vi "FreqPeakFit.vi"(6 "error in (no error)":errorcluster, 8 "Peak fit width":i32=3 min=3, 9 "Waveform":waveform(dbl)={"t0"=timestamp(0.1098 s since 1904-01-01), "dt"=1e-07, "Y"=array[1000 elements], "attributes"=variant("Channel_name"=variant(string "CH1"), "NI_ChannelName"=variant(string "CH1"), "Total_points"=variant(i64 1200000))}) -> (0 "error out":errorcluster, 2 "Amplitude":dbl, 3 "PeakFreqOut":dbl)   [LabVIEW 2019]
uses:
  <vilib>/measure/mamon.llb/Waveform Peak Detection for 1 Chan.vi
  <vilib>/measure/NI_MAPro.lvlib
panel:
  out "Freq3":dbl
  out "Freq2":dbl
  out "Freq":dbl
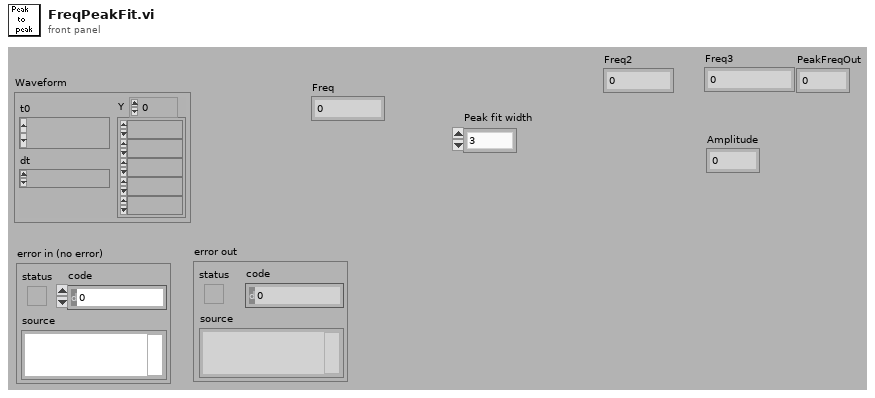
[diagram p1: front panel]
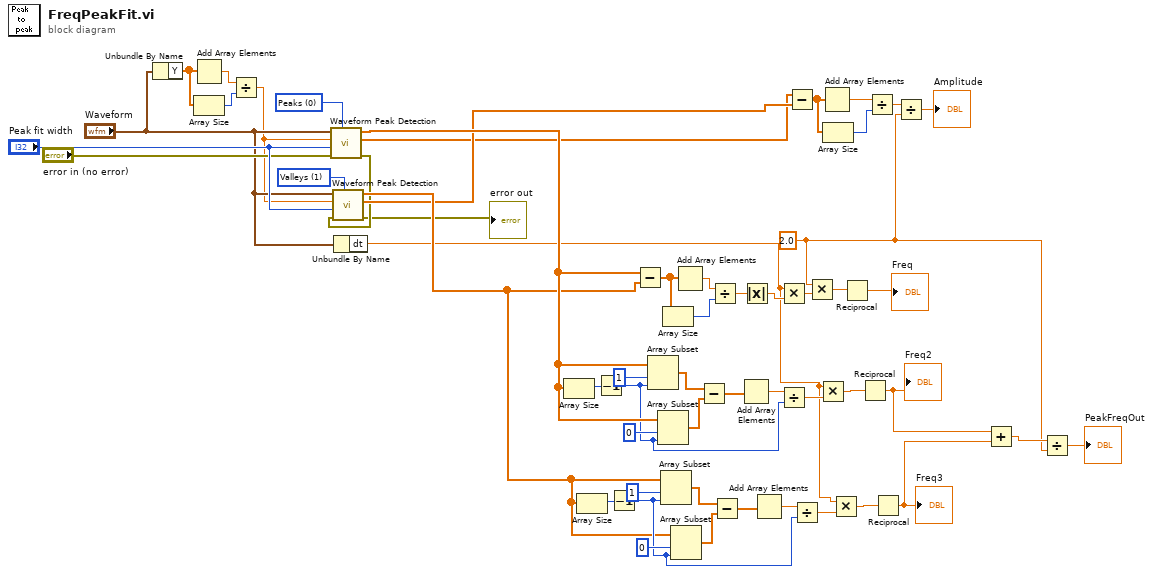
[diagram p0: block diagram]
diagram:
  w10 = u16 0 items=["Peaks", "Valleys"] ("peaks/valleys")
  w11 = 2.0
  w54 = u16 1 items=["Peaks", "Valleys"] ("peaks/valleys")
  n1 = Unbundle By Name("Waveform") -> ("Y"=w4:dbl[])
  n2 = Add Array Elements(numeric array=w4) -> (sum=w2:dbl)
  n3 = Array Size(array=w4) -> (size(s)=w3:i32)
  n4 = Divide(x=w2, y=w3) -> (x/y=w1:dbl)
  n5 = call-poly <vilib>:"Waveform Peak Detection.vi"("peaks/valleys"=w10, "error in"="error in (no error)", "width"="Peak fit width", "threshold"=w1, "Signal In"="Waveform") -> ("error out"=w7:errorcluster, "Amplitudes"=w14:dbl[], "Locations"=w39:dbl[])  [unwired: 2 in, 2 out]
  n6 = call-poly <vilib>:"Waveform Peak Detection.vi"("peaks/valleys"=w54, "error in"=w7, "width"="Peak fit width", "threshold"=w1, "Signal In"="Waveform") -> ("error out"=→"error out":errorcluster, "Amplitudes"=w18:dbl[], "Locations"=w19:dbl[])  [unwired: 2 in, 2 out]
  n7 = Unbundle By Name("Waveform") -> ("dt"=w9:dbl)
  n8 = Array Size(array=w39) -> (size(s)=w44:i32)
  n9 = Array Size(array=w19) -> (size(s)=w33:i32)
  n10 = Decrement(x=w44) -> (x-1=w36:i32)
  n11 = Decrement(x=w33) -> (x-1=w26:i32)
  n12 = Subtract(x=w39, y=w19) -> (x-y=w51:dbl[])
  n13 = Array Subset(array=w39, index=1, length=w36) -> (w41:dbl[])
  n14 = Array Subset(array=w39, index=0, length=w36) -> (w40:dbl[])
  n15 = Array Subset(array=w19, index=1, length=w26) -> (w30:dbl[])
  n16 = Array Size(array=w51) -> (size(s)=w49:i32)
  n17 = Array Subset(array=w19, index=0, length=w26) -> (w29:dbl[])
  n18 = Add Array Elements(numeric array=w51) -> (sum=w52:dbl)
  n19 = Subtract(x=w41, y=w40) -> (x-y=w38:dbl[])
  n20 = Divide(x=w52, y=w49) -> (x/y=w50:dbl)
  n21 = Subtract(x=w30, y=w29) -> (x-y=w28:dbl[])
  n22 = Add Array Elements(numeric array=w38) -> (sum=w37:dbl)
  n23 = Absolute Value(x=w50) -> (abs(x)=w48:dbl)
  n24 = Add Array Elements(numeric array=w28) -> (sum=w27:dbl)
  n25 = Multiply(x=w9, y=w48) -> (x*y=w47:dbl)
  n26 = Divide(x=w37, y=w36) -> (x/y=w35:dbl)
  n27 = Subtract(x=w14, y=w18) -> (x-y=w15:dbl[])
  n28 = Divide(x=w27, y=w26) -> (x/y=w25:dbl)
  n29 = Multiply(x=w11, y=w47) -> (x*y=w46:dbl)
  n30 = Multiply(x=w9, y=w35) -> (x*y=w34:dbl)
  n31 = Add Array Elements(numeric array=w15) -> (sum=w17:dbl)
  n32 = Array Size(array=w15) -> (size(s)=w16:i32)
  n33 = Multiply(x=w9, y=w25) -> (x*y=w24:dbl)
  n34 = Reciprocal(x=w46) -> (1/x=→"Freq":dbl)
  n35 = Reciprocal(x=w34) -> (1/x=w23:dbl)
  "Freq2" <- w23
  n36 = Divide(x=w17, y=w16) -> (x/y=w12:dbl)
  n37 = Reciprocal(x=w24) -> (1/x=w22:dbl)
  "Freq3" <- w22
  n38 = Divide(x=w12, y=w11) -> (x/y=→"Amplitude":dbl)
  n39 = Add(x=w23, y=w22) -> (x+y=w21:dbl)
  n40 = Divide(x=w21, y=w11) -> (x/y=→"PeakFreqOut":dbl)
